vi "Encoder-Calibration.vi"   [LabVIEW 2016, in "LEGO-PMR.lvrbt"]
uses:
  LEGO-PMR.lvrbt
  <vilib>/NXT/Block Support/NXT_OutputPort.ctl
  <vilib>/NXT/NXTIO Xnodes/NXTIONodeSubVIs/LEGOResetMotors.vi
  <vilib>/NXT/NXTIO Xnodes/NXTIONodeSubVIs/NXTMotorRunDistance.vi
  <vilib>/NXT/NXTIO Xnodes/AddressXNode/NXTIOAddress.xnode
  <vilib>/NXT/Subs/LVHSConnector.ctl
  <vilib>/NXT/NXTIO Xnodes/NXTIOXNode/NXTIO.xnode
  <vilib>/NXT/LegoClasses/BrickReference/BrickReference.lvclass
types:
  T1 = typedef "NXT_OutputPort.ctl" = u8
  T2 = typedef "LVHSConnector.ctl" = refnum<class "BrickReference.lvclass">
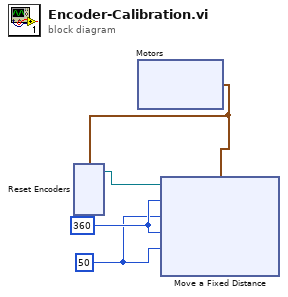
[diagram p0: block diagram]
diagram:
  w1 = 50
  w2 = 360
  n1 = xnode "Motors"() -> ("Motor"=w3:cluster{"Port":T1, "Port":T1})
  n2 = xnode "Reset Encoders"("Motors"=w3) -> ("NXT/EV3"=w4:T2)  [unwired: 1 in]
  n3 = xnode "Move a Fixed Distance"("Speed 2"=w1, "Speed 1"=w1, "Distance 2"=w2, "Distance 1"=w2, "Motors"=w3, "NXT/EV3"=w4) -> ()  [unwired: 1 in, 1 out]
